vi "Merge Sensors.vi"(0 "Source Sensors IN":T1[](array[typedef]) {"Max Error % of Reading" format="%.2f"; "Max Stability Error" format="%.2f"; "Max Mean Squared Error" format="%.2f"; "Max Error % of Full Scale" format="%.2f"; "Coefficients" format="%.2f"; "Voltage List" format="%.2f"; "EGU List" format="%.2f"; "EGU Range"."Low Limit" format="%.2f"; "EGU Range"."High Limit" format="%.2f"; "Voltage Range"."Low Limit" format="%.2f"; "Voltage Range"."High Limit" format="%.2f"; "Last Cal Info"."Last Calibration Date" format="%.2f"}, 1 "Server is Source (T)":bool=TRUE, 5 "Dest Sensors IN":T1[](array[typedef]) {"Max Error % of Reading" format="%.2f"; "Max Stability Error" format="%.2f"; "Max Mean Squared Error" format="%.2f"; "Max Error % of Full Scale" format="%.2f"; "Coefficients" format="%.2f"; "Voltage List" format="%.2f"; "EGU List" format="%.2f"; "EGU Range"."Low Limit" format="%.2f"; "EGU Range"."High Limit" format="%.2f"; "Voltage Range"."Low Limit" format="%.2f"; "Voltage Range"."High Limit" format="%.2f"; "Last Cal Info"."Last Calibration Date" format="%.2f"}, 11 "Error IN":errorcluster, 12 "Version Prompt (F)":bool) -> (4 "Source Sensors OUT":T1[](array[typedef]) {"Max Error % of Reading" format="%.2f"; "Max Stability Error" format="%.2f"; "Max Mean Squared Error" format="%.2f"; "Max Error % of Full Scale" format="%.2f"; "Coefficients" format="%.2f"; "Voltage List" format="%.2f"; "EGU List" format="%.2f"; "EGU Range"."Low Limit" format="%.2f"; "EGU Range"."High Limit" format="%.2f"; "Voltage Range"."Low Limit" format="%.2f"; "Voltage Range"."High Limit" format="%.2f"; "Last Cal Info"."Last Calibration Date" format="%.2f"}, 6 "Dest Sensors OUT":T1[](array[typedef]) {"Max Error % of Reading" format="%.2f"; "Max Stability Error" format="%.2f"; "Max Mean Squared Error" format="%.2f"; "Max Error % of Full Scale" format="%.2f"; "Coefficients" format="%.2f"; "Voltage List" format="%.2f"; "EGU List" format="%.2f"; "EGU Range"."Low Limit" format="%.2f"; "EGU Range"."High Limit" format="%.2f"; "Voltage Range"."Low Limit" format="%.2f"; "Voltage Range"."High Limit" format="%.2f"; "Last Cal Info"."Last Calibration Date" format="%.2f"}, 8 "Source Changed":bool, 10 "Dest Changed":bool, 15 "Error OUT":errorcluster)   [LabVIEW 2023]
uses:
  Type Defs and Controls/Sensor.ctl
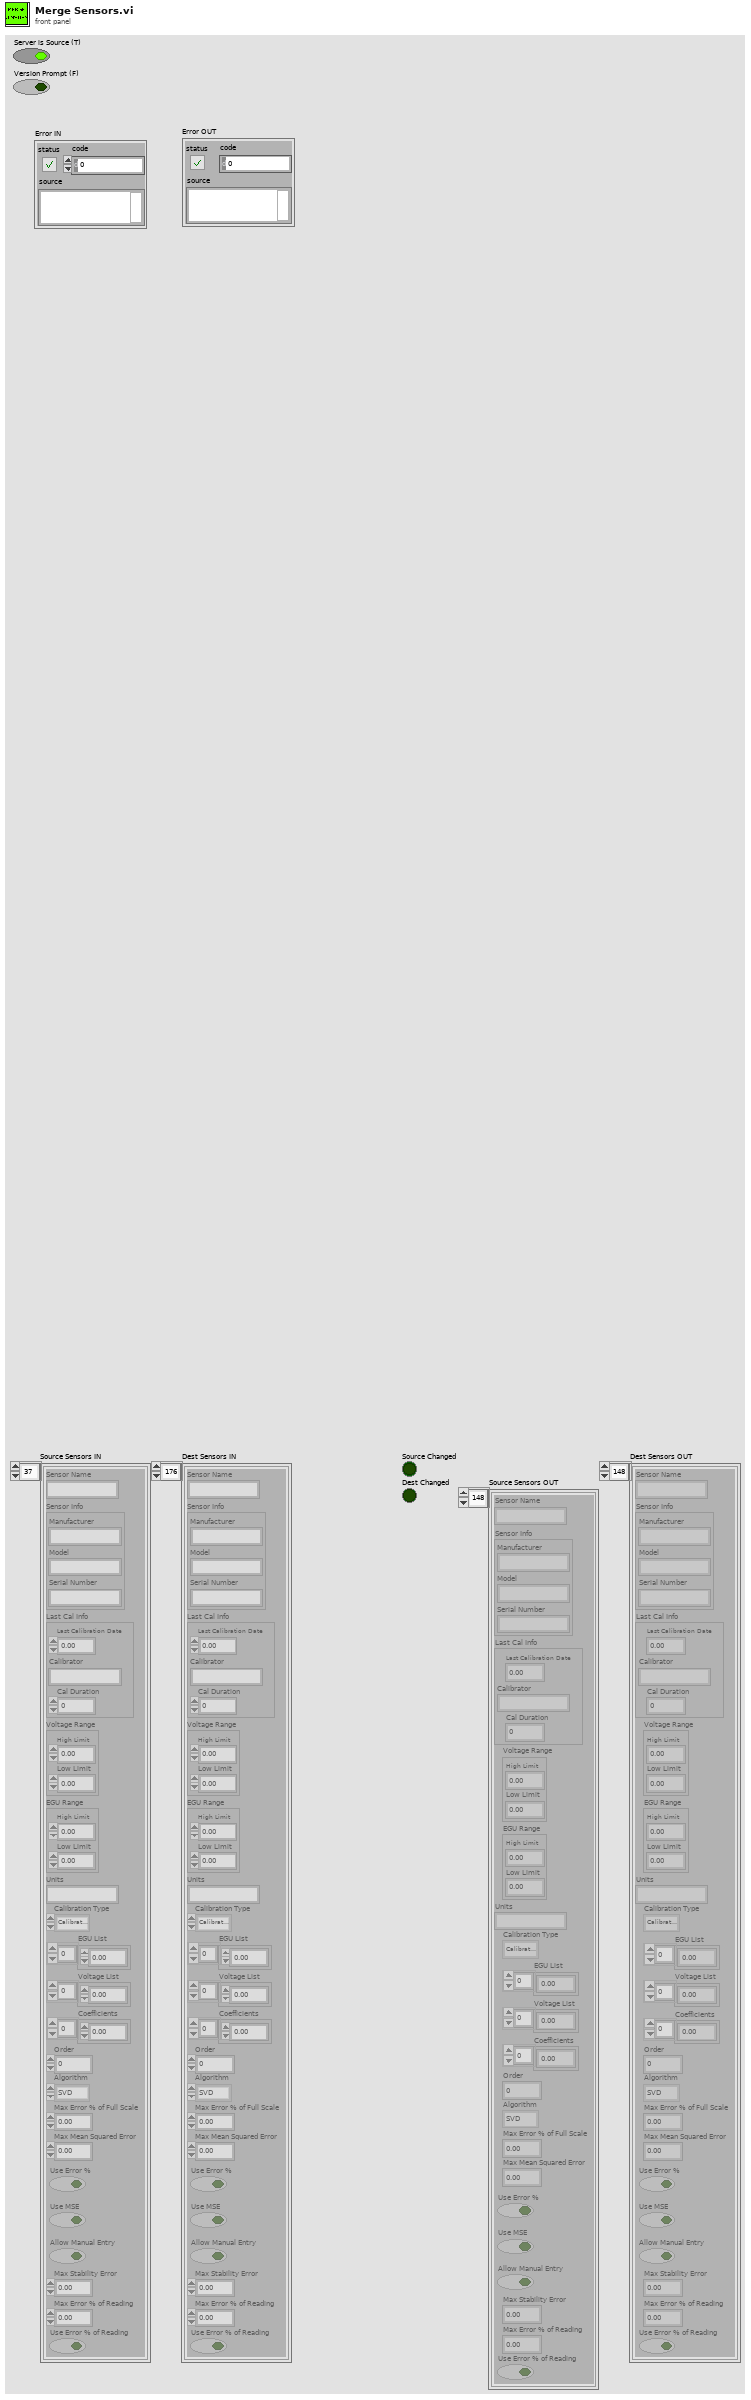
[diagram p1: front panel]
types:
  T1 = typedef "Sensor.ctl" = cluster{"Sensor Name":string, "Sensor Info":cluster{"Manufacturer":string, "Model":string, "Serial Number":string}, "Last Cal Info":cluster{"Last Calibration Date":dbl, "Calibrator":string, "Cal Duration":i32}, "Voltage Range":cluster{"High Limit":dbl, "Low Limit":dbl}, "EGU Range":cluster{"High Limit":dbl, "Low Limit":dbl}, "Units":string, "Calibration Type":enum16{"Calibrate Analog", "Compare Analog Calibration"}, "EGU List":dbl[], "Voltage List":dbl[], "Coefficients":dbl[], "Order":i32, "Algorithm":enum32{"SVD", "Givens", "Givens2", "Householder", "LU Decomposition", "Cholesky"}, "Max Error % of Full Scale":dbl, "Max Mean Squared Error":dbl, "Use Error %":bool, "Use MSE":bool, "Allow Manual Entry":bool, "Max Stability Error":dbl, "Max Error % of Reading":dbl, "Use Error % of Reading":bool}
  T2 = enum16{"Left Button", "Center Button", "Right Button", "Window Close"}
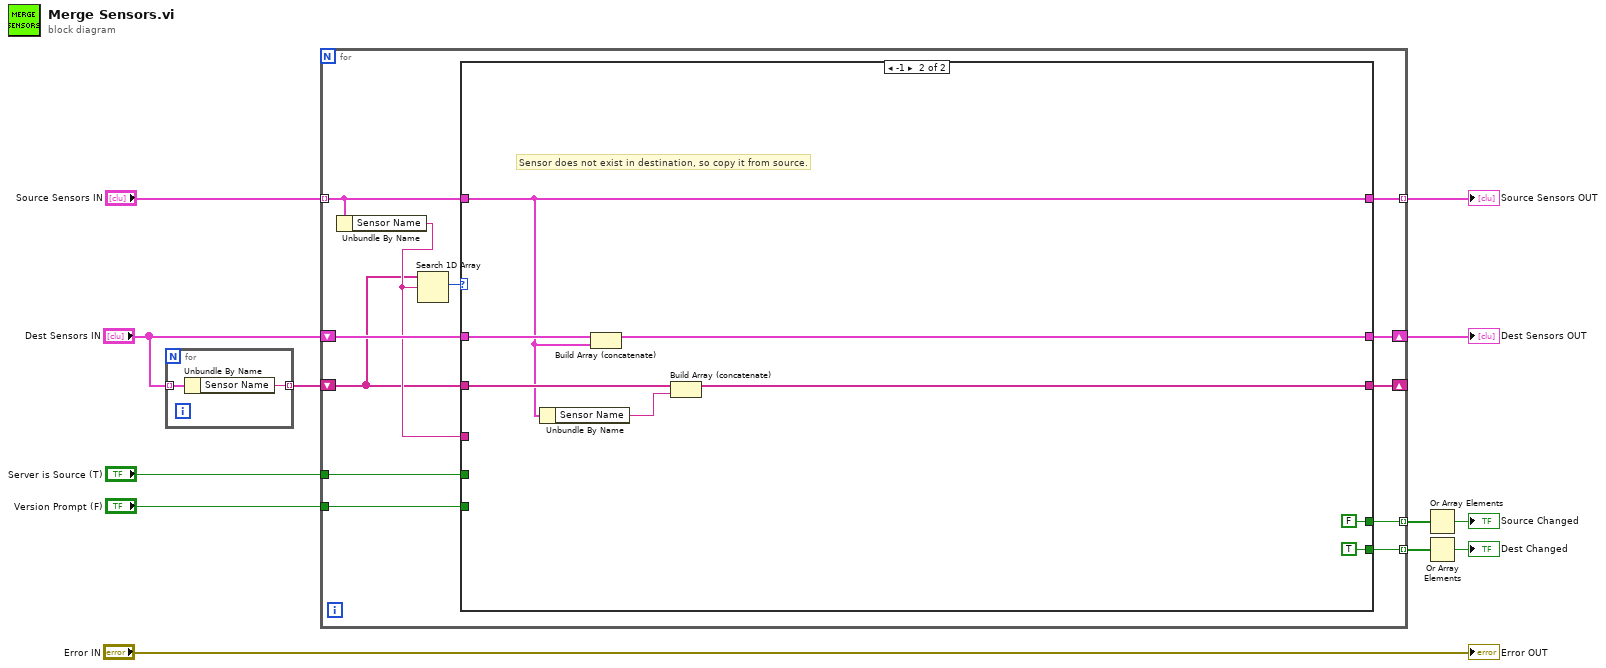
[diagram p0: block diagram]
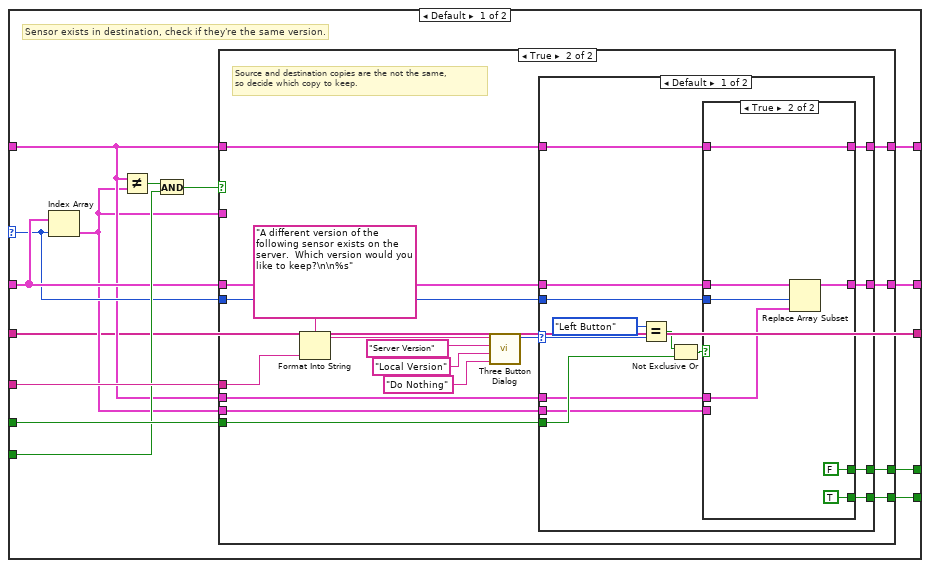
[diagram p2: hidden frame]
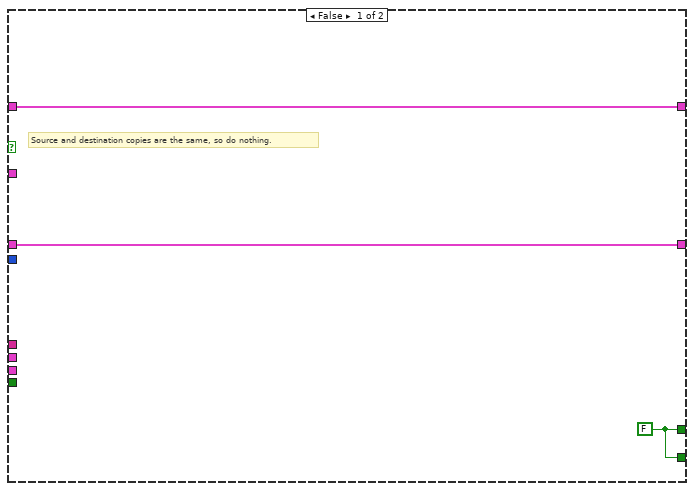
[diagram p3: hidden frame]
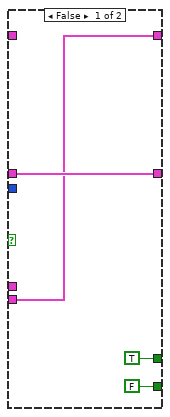
[diagram p4: hidden frame]
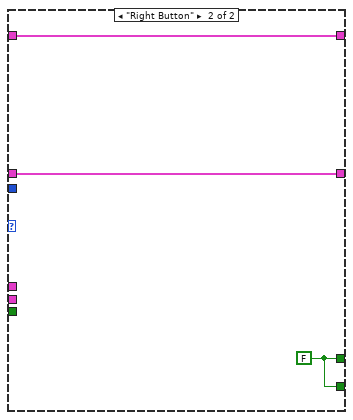
[diagram p5: hidden frame]
diagram:
  n1 = for {
    tunnel: "Dest Sensors IN" -> [w14] mode=indexing
    tunnel: [w13] -> w1 mode=indexing
    n2 = Unbundle By Name(w14) -> ("Sensor Name"=w13:string)
  }
  n3 = for {
    tunnel: "Server is Source (T)" -> [w25]
    tunnel: "Version Prompt (F)" -> [w24]
    shift-right: [w22] -> w4
    shift-left: "Dest Sensors IN" -> [w23]
    tunnel: [w21] -> w8 mode=indexing
    tunnel: [w20] -> w5 mode=indexing
    tunnel: "Source Sensors IN" -> [w18] mode=indexing
    tunnel: [w19] -> w2 mode=indexing
    shift-right: [w15] -> _
    shift-left: w1 -> [w16]
    n4 = Unbundle By Name(w18) -> ("Sensor Name"=w17:string)
    n5 = Search 1D Array(1D array=w16, element=w17) -> (index of element=w26:i32)  [unwired: 1 in]
    n6 = case shown="-1" w26 {
      selector: w26 -> [w33 _]
      tunnel: w17 -> [w40 _]
      tunnel: w25 -> [w39 _]
      tunnel: w24 -> [w37 _]
      tunnel: w23 -> [w34 w96]
      tunnel: [w32 w95] -> w22
      tunnel: [w35 w91] -> w19
      tunnel: [w31 FALSE ("Source Changed")] -> w21
      tunnel: [w30 TRUE ("Source Changed")] -> w20
      tunnel: w18 -> [w29 w91]
      tunnel: w16 -> [w27 w92]
      tunnel: [w27 w89] -> w15
      frame Default {
        # "Sensor exists in destination, check if they're the same version."
        n7 = Index Array(array=w34, index=w33) -> (element=w28:T1)
        n8 = Not Equal?(x=w29, y=w28) -> (x != y?=w38:bool)
        n9 = And(x=w38, y=w37) -> (x .and. y?=w36:bool)
        n10 = case shown="True" w36 {
          tunnel: w40 -> [_ w60]
          tunnel: w39 -> [_ w58]
          tunnel: w29 -> [_ w57]
          tunnel: w28 -> [_ w56]
          tunnel: w29 -> [w43 w44]
          tunnel: [w43 w50] -> w35
          tunnel: w34 -> [w42 w49]
          tunnel: w33 -> [_ w48]
          tunnel: [w42 w47] -> w32
          tunnel: [w41 w46] -> w31
          tunnel: [w41 w45] -> w30
          tunnel: w28 -> [_ _]
          frame False {
            w41 = FALSE ("Source Changed")
            # "Source and destination copies are the same, so do nothing."
          }
          frame True {
            # "Source and destination copies are the not the same,\nso decide which copy to keep."
            n11 = Format Into String(format string="A different version of the following sensor exists on the server.  Which version would you like to keep?\n\n%s" ("message"), w60) -> (resulting string=w59:string)  [unwired: 2 in, 1 out]
            n12 = call <vilib>:"Three Button Dialog.vi"("Right Button Text (\"Cancel\")"="Do Nothing" ("T button name (\"OK\")"), "Center Button Text (\"No\")"="Local Version" ("T button name (\"OK\")"), "Left Button Text (\"Yes\")"="Server Version" ("T button name (\"OK\")"), "message"=w59) -> ("Which Button?"=w51:T2)  [unwired: 7 in]
            n13 = case shown="Default" w51 {
              selector: w51 -> [w70 _]
              tunnel: w58 -> [w74 _]
              tunnel: w57 -> [w72 _]
              tunnel: w56 -> [w71 _]
              tunnel: w44 -> [w67 w88]
              tunnel: [w66 w88] -> w50
              tunnel: w49 -> [w65 w87]
              tunnel: w48 -> [w64 _]
              tunnel: [w63 w87] -> w47
              tunnel: [w62 w86] -> w46
              tunnel: [w61 w86] -> w45
              frame Default {
                n14 = Equal?(x=T2."Left Button", y=w70) -> (x = y?=w68:bool)
                n15 = Not Exclusive Or(1:w74, 2:w68) -> (0:w73:bool)
                n16 = case shown="True" w73 {
                  tunnel: w72 -> [_ w82]
                  tunnel: w71 -> [w75 _]
                  tunnel: w67 -> [_ w85]
                  tunnel: [w75 w85] -> w66
                  tunnel: w65 -> [w78 w84]
                  tunnel: w64 -> [_ w83]
                  tunnel: [w78 w81] -> w63
                  tunnel: [TRUE ("Source Changed") FALSE ("Source Changed")] -> w62
                  tunnel: [FALSE ("Source Changed") TRUE ("Source Changed")] -> w61
                  frame False {
                  }
                  frame True {
                    n17 = Replace Array Subset(array=w84, new element=w82, index=w83) -> (w81:T1[])
                  }
                }
              }
              frame "Right Button" {
                w86 = FALSE ("Source Changed")
              }
            }
          }
        }
      }
      frame -1 {
        # "Sensor does not exist in destination, so copy it from source."
        n18 = Unbundle By Name(w91) -> ("Sensor Name"=w90:string)
        n19 = Build Array (concatenate)(w96, w91) -> (w95:T1[])
        n20 = Build Array (concatenate)(w92, w90) -> (w89:string[])
      }
    }
  }
  "Source Sensors OUT" <- w2
  "Dest Sensors OUT" <- w4
  n21 = Or Array Elements(Boolean array=w8) -> (logical OR=→"Source Changed":bool)
  n22 = Or Array Elements(Boolean array=w5) -> (logical OR=→"Dest Changed":bool)
  "Error OUT" <- "Error IN"
